vi "Separator.vi"() -> (0 "Separator":string="$$$")   [LabVIEW 2020, in "Caraya.lvlib" / "Basic Test Manager.lvclass"]
uses:
  Basic Test Manager.lvclass
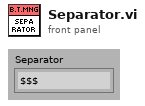
[diagram p1: front panel]
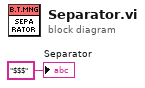
[diagram p0: block diagram]
diagram:
  "Separator" <- "$$$"
